vi "_Main_ByRuns_DAC2022.vi"() -> ()   [LabVIEW 2017]
uses:
  <vilib>/Instr/_visa.llb/VISA Configure Serial Port (Instr).vi
panel:
  out "Field, kV/cm":dbl
  out "Current, mA":dbl
  out "Voltage, V":dbl
  in  "COM DAC":refnum<visa-resource-name>
  in  "WaveForm":i32(listbox)
  in  "Auto\nturn OFF":bool
  in  "Content":i32(listbox)
  out "LastTrigTimer, s":dbl
  in  "Graph every, cycle":dbl=10.0 min=1.0 max=100.0
  in  "SendPeriod, ms":dbl=100.0 min=10.0 max=10000.0
  out "RunsNeed":i32
  out "Time LOG":cluster{dbl[], dbl[]}(graph)
  out "LED2":bool
  out "LED1":bool
  out "TrigTimer, s":dbl
  out "Bytes at Port":u32
  out "RecTry":i32
  out "OutVoltage, V":dbl
  in  "Exposition, s":dbl=3.0
  out "Channel 2, V":dbl format="%#_5g"
  out "Channel 1, V":dbl format="%#_5g"
  in  "Stop Button":bool
  in  "Start Button":bool
  in  "Sample H, um":dbl=32.0
  out "VoltageArray, V":dbl[](array[numeric])
  out "Shutter Red":bool
  out "Shutter Green":bool
  in  "Frames In Run":u32=180
  out "Global Frame Done":u32
  out "Now is Run #":u32
  out "Frame In Run Done":u32
  in  "Step, kV/cm":dbl=1.0 min=0.01 max=1000.0
  in  "Amplitude, kV/cm":dbl=10.0 min=10.0 max=1500.0
  in  "LOG file":path
  in  "COM ADC":refnum<visa-resource-name>
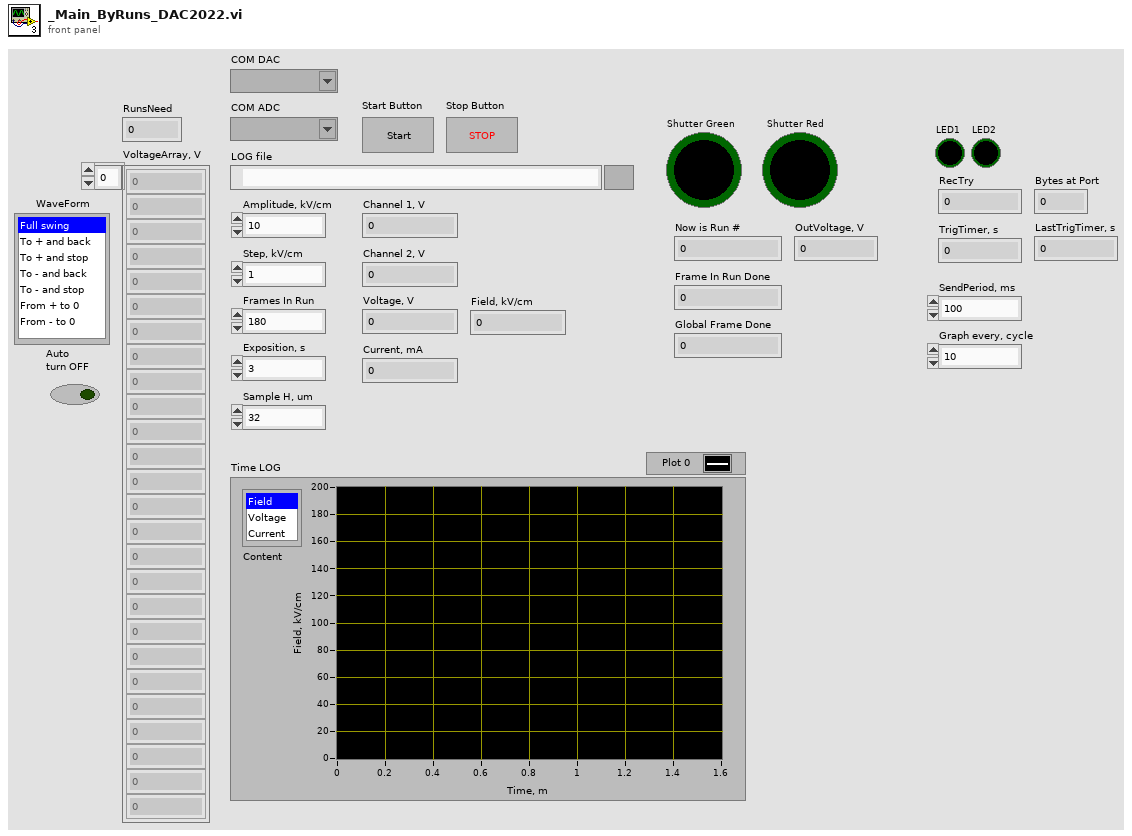
[diagram p1: front panel]
types:
  T1 = cluster{i32, i32, u32, "TrigState":bool, "TrigTimer, s":dbl, "CurrentError":bool}
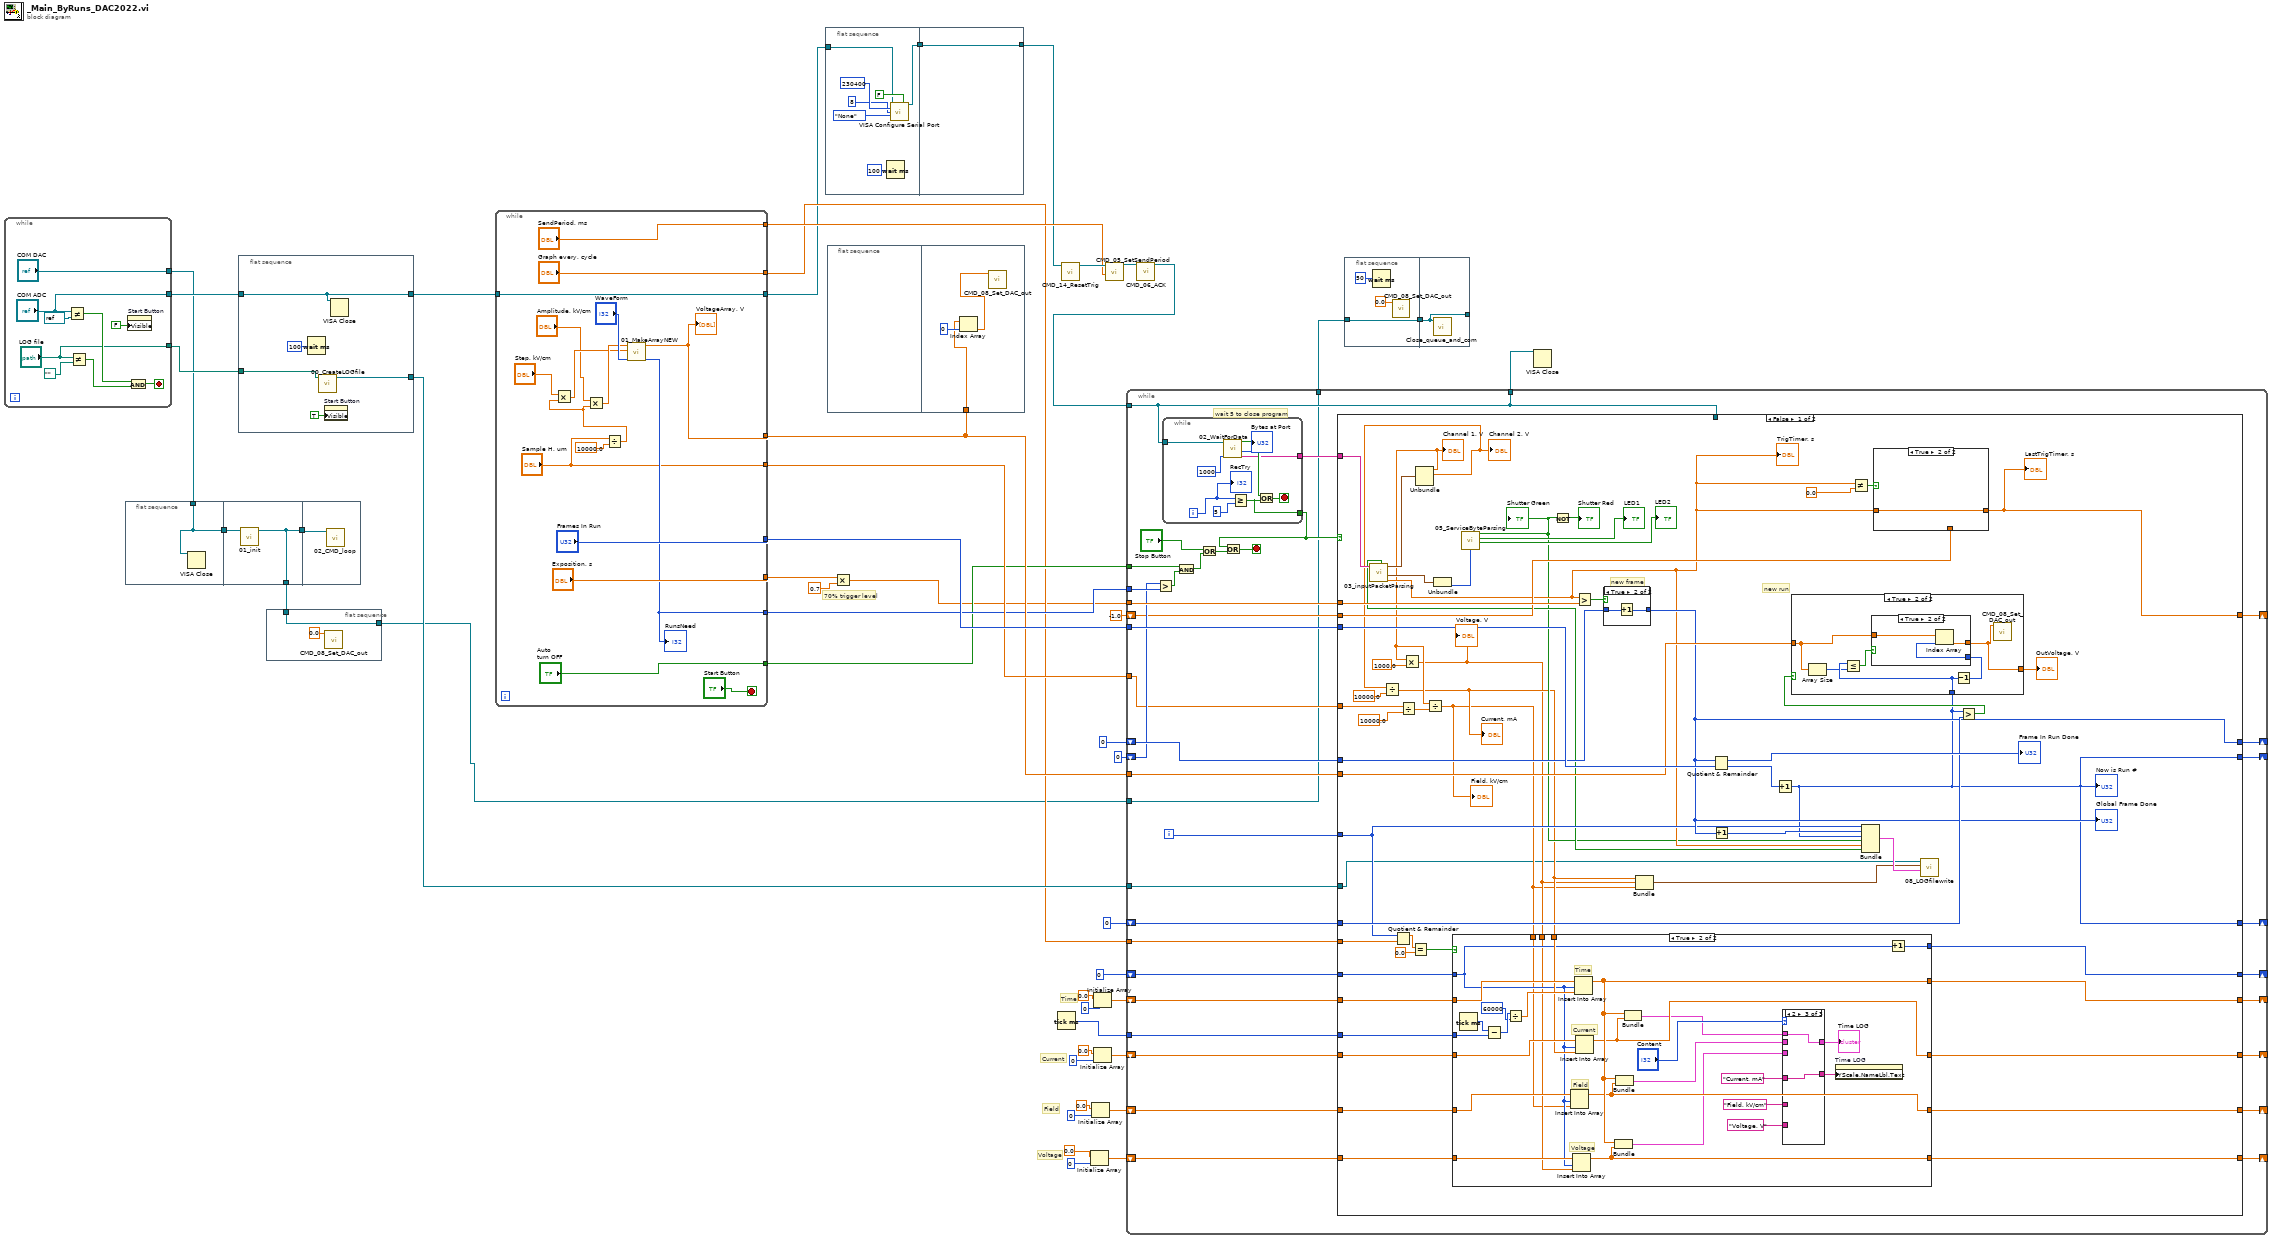
[diagram p0: block diagram]
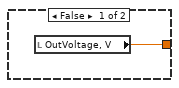
[diagram p6: hidden frame]
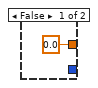
[diagram p7: hidden frame]
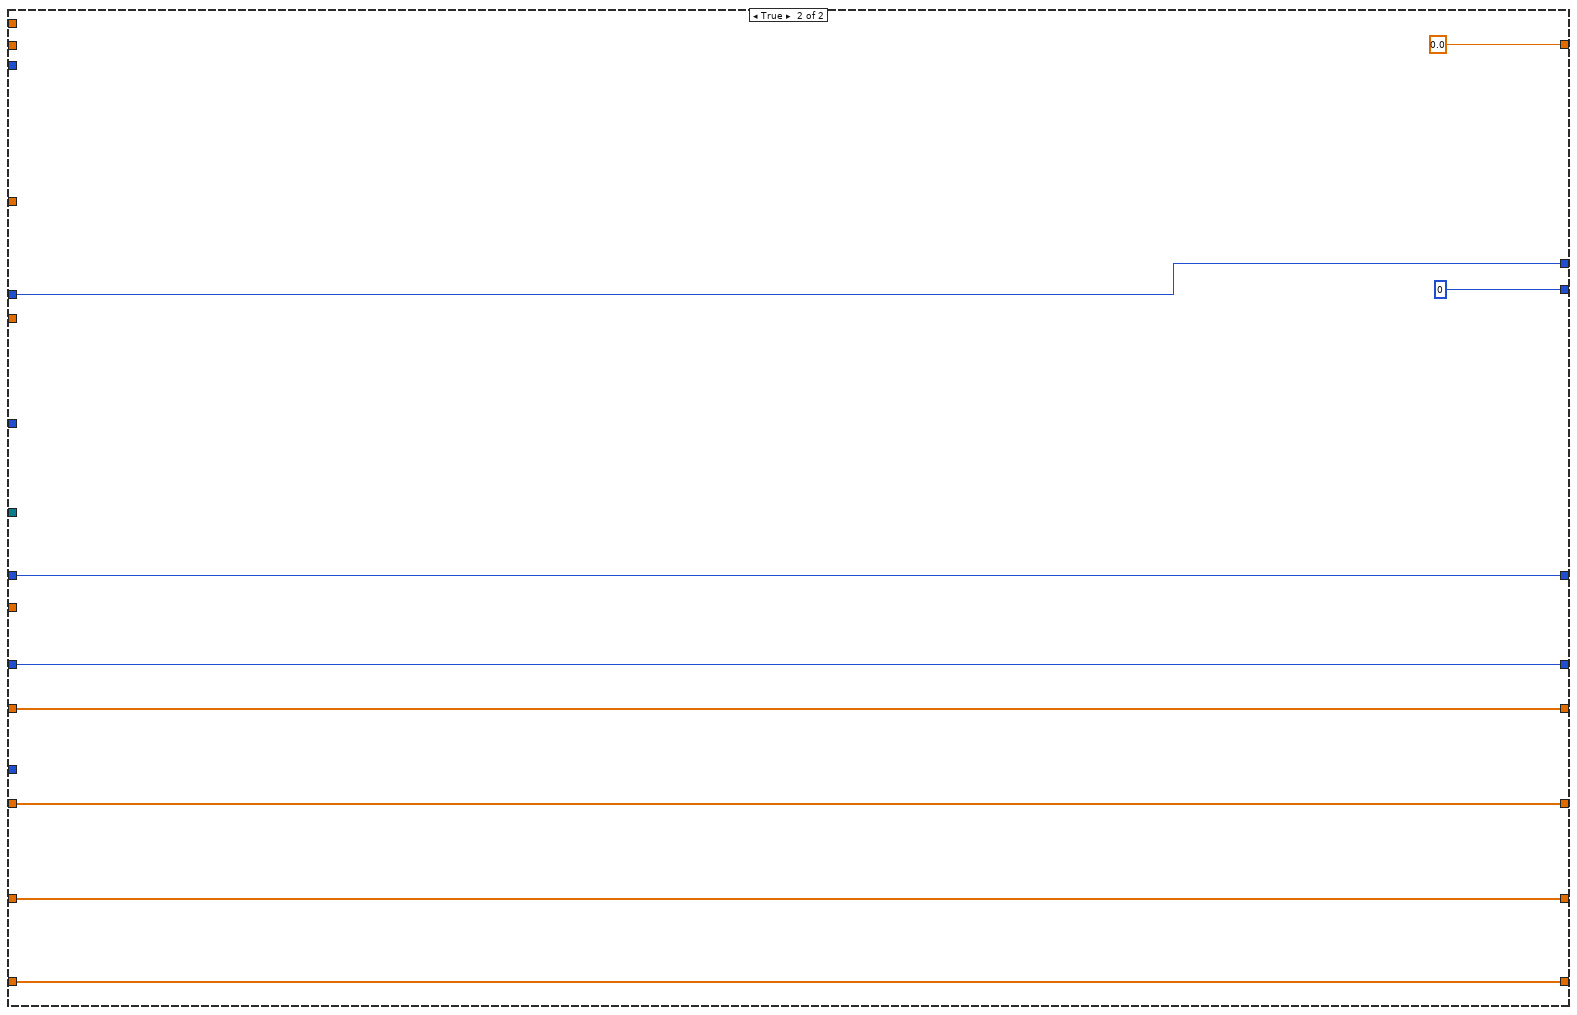
[diagram p9: hidden frame]
diagram:
  # "70% trigger level"
  # "Voltage"
  # "Field"
  # "Time"
  # "Current"
  n1 = while {
    tunnel: ["COM ADC"] -> w14
    tunnel: ["LOG file"] -> w13
    tunnel: ["COM DAC"] -> w5
    stop <- w53 stop-if-true
    n2 = Not Equal?(x="COM ADC", y=refnum<visa-resource-name> refnum ("COM port")) -> (x != y?=w50:bool)
    n3 = Not Equal?(x="LOG file", y=path "" ("LOG file")) -> (x != y?=w51:bool)
    n4 = property on="Start Button" class="Bool"("Visible"=FALSE) -> ()  [unwired: 2 in, 2 out]
    n5 = And(x=w50, y=w51) -> (x .and. y?=w53:bool)
  }
  n6 = flat-sequence {
    tunnel: [w56] -> w7
    tunnel: w5 -> [w56]
    tunnel: w7 -> [w58]
    tunnel: [w57] -> w4
    tunnel: [w57] -> w6
    tunnel: w6 -> [w59]
    frame #0 {
      n7 = VISA Close(VISA resource name=w56) -> ()  [unwired: 1 in, 1 out]
    }
    frame #1 {
      n8 = call "01_init.vi"("COM port"=w58) -> ("VISA resource name out"=w57:refnum<visa-resource-name>)  [unwired: 8 in, 2 out]
    }
    frame #2 {
      n9 = call "02_CMD_loop.vi"("VISA resource name"=w59) -> ()  [unwired: 11 in]
    }
  }
  n10 = flat-sequence {
    tunnel: [w64] -> w44
    tunnel: w14 -> [w60]
    tunnel: w13 -> [w61]
    tunnel: [w60] -> w12
    frame #0 {
      n11 = Wait (ms)(milliseconds to wait=u32 100) -> ()  [unwired: 1 out]
      n12 = call "00_CreateLOGfile.vi"("LOG file"=w61) -> ("refnum out"=w64:refnum<file>)  [unwired: 10 in]
      n13 = property on="Start Button" class="Bool"("Visible"=TRUE) -> ()  [unwired: 2 in, 2 out]
      n14 = VISA Close(VISA resource name=w60) -> ()  [unwired: 1 in, 1 out]
    }
  }
  n15 = flat-sequence {
    tunnel: w4 -> [w65]
    tunnel: [w65] -> w1
    frame #0 {
      n16 = call "CMD_08_Set_DAC_out.vi"("DAC voltage, V"=0.0) -> ()  [unwired: 11 in]
    }
  }
  n17 = while {
    tunnel: w12 -> [w76]
    tunnel: [w76] -> w10
    tunnel: [w75] -> w38
    tunnel: ["Sample H, um"] -> w45
    tunnel: ["Frames In Run"] -> w46
    tunnel: ["Exposition, s"] -> w23
    tunnel: [w74] -> w29
    tunnel: ["Auto\nturn OFF"] -> w27
    tunnel: ["SendPeriod, ms"] -> w26
    tunnel: ["Graph every, cycle"] -> w25
    stop <- "Start Button" stop-if-true
    n18 = Divide(x="Sample H, um", y=10000.0) -> (x/y=w68:dbl)
    n19 = Multiply(x="Step, kV/cm", y=w68) -> (x*y=w70:dbl)
    n20 = Multiply(x="Amplitude, kV/cm", y=w68) -> (x*y=w71:dbl)
    n21 = call "01_MakeArrayNEW.vi"("Amp"=w71, "Step"=w70, "WaveForm"="WaveForm") -> ("Array"=w75:dbl[], "ArraySize"=w74:i32)  [unwired: 6 in]
    "VoltageArray, V" <- w75
    "RunsNeed" <- w74
  }
  n22 = flat-sequence {
    tunnel: w10 -> [w86]
    tunnel: [w85] -> w11
    tunnel: w11 -> [w91]
    tunnel: [w91] -> w9
    frame #0 {
      n23 = Wait (ms)(milliseconds to wait=u32 100) -> ()  [unwired: 1 out]
      n24 = call-poly "VISA Configure Serial Port"("VISA resource name"=w86, "Enable Termination\nChar (T)"=FALSE ("Enable Termination\nChar (T)"), "baud rate (9600)"=u32 230400, "data bits (8)"=u16 8, "parity (0:none)"=enum16{"None", "Odd", "Even", "Mark", "Space"}."None") -> ("VISA resource name out"=w85:refnum<visa-resource-name>)  [unwired: 9 in, 1 out]
    }
    frame #1 {
    }
  }
  n25 = flat-sequence {
    tunnel: w38 -> [w93]
    frame #0 {
    }
    frame #1 {
      n26 = Index Array(array=w93, index=0) -> (element=w92:dbl)
      n27 = call "CMD_08_Set_DAC_out.vi"("DAC voltage, V"=w92) -> ()  [unwired: 11 in]
    }
  }
  n28 = Multiply(x=w23, y=0.7) -> (x*y=w24:dbl)
  n29 = Tick Count (ms)() -> (millisecond timer value=w33:u32)
  n30 = call "CMD_14_ResetTrig.vi"("VISA resource name"=w9) -> ("VISA resource name out"=w41:refnum<visa-resource-name>)  [unwired: 10 in]
  n31 = Initialize Array(0.0 ("element"), 0 ("dimension size")) -> (w15:dbl[])
  n32 = Initialize Array(0.0 ("element"), 0 ("dimension size")) -> (w16:dbl[])
  n33 = Initialize Array(0.0 ("element"), 0 ("dimension size")) -> (w30:dbl[])
  n34 = Initialize Array(0.0 ("element"), 0 ("dimension size")) -> (w34:dbl[])
  n35 = call "CMD_05_SetSendPeriod.vi"("Period, ms"=w26, "VISA resource name"=w41) -> ("VISA resource name out"=w40:refnum<visa-resource-name>)  [unwired: 9 in]
  n36 = call "CMD_06_ACK.vi"("VISA resource name"=w40) -> ("VISA resource name out"=w39:refnum<visa-resource-name>)  [unwired: 10 in]
  n37 = while {
    tunnel: w39 -> [w96]
    tunnel: w38 -> [w120]
    tunnel: w46 -> [w126]
    tunnel: w24 -> [w128]
    tunnel: w45 -> [w97]
    tunnel: w44 -> [w127]
    shift-right: [w123] -> _
    shift-left: 0 -> [w125]
    shift-right: [w122] -> _
    shift-left: u32 0 -> [w121]
    shift-right: [w118] -> _
    shift-left: 0 -> [w119]
    tunnel: w33 -> [w116]
    shift-right: [w114] -> _
    shift-left: w34 -> [w117]
    shift-right: [w113] -> _
    shift-left: w30 -> [w115]
    tunnel: w29 -> [w109]
    shift-right: [w111] -> _
    shift-left: u32 0 -> [w108]
    tunnel: w27 -> [w105]
    tunnel: w25 -> [w104]
    shift-right: [w103] -> _
    shift-left: -1.0 ("TrigTimer, s") -> [w102]
    shift-right: [w99] -> _
    shift-left: w16 -> [w101]
    shift-right: [w98] -> _
    shift-left: w15 -> [w100]
    tunnel: [w95] -> w2
    tunnel: [w96] -> w8
    tunnel: w1 -> [w95]
    i -> [w124]
    stop <- w131 stop-if-true
    # "wait 5 to close program"
    n38 = Greater?(x=w108, y=w109) -> (0:w106:bool)
    n39 = while {
      tunnel: w96 -> [w251]
      tunnel: [w254] -> w130
      tunnel: [w255] -> w129
      i -> [w253]
      stop <- w257 stop-if-true
      n40 = call "02_WaitForData.vi"("WaitTimeoutMS"=u32 1000, "VISA"=w251) -> ("Buffer"=w255:string, "Bytes at Port"=→"Bytes at Port":u32, "Data Recived"=w256:bool)  [unwired: 7 in]
      n41 = Greater Or Equal?(x=w253, y=5) -> (x >= y?=w254:bool)
      n42 = Or(x=w256, y=w254) -> (x .or. y?=w257:bool)
      "RecTry" <- w253
    }
    n43 = And(x=w105, y=w106) -> (x .and. y?=w107:bool)
    n44 = Or(x="Stop Button", y=w107) -> (x .or. y?=w112:bool)
    n45 = Or(x=w130, y=w112) -> (x .or. y?=w131:bool)
    n46 = case shown="False" w130 {
      tunnel: w129 -> [w187 _]
      tunnel: w128 -> [w183 _]
      tunnel: w127 -> [w132 _]
      tunnel: w126 -> [w184 _]
      tunnel: w125 -> [w181 w250]
      tunnel: w124 -> [w166 _]
      tunnel: [w173 w250] -> w123
      tunnel: [w157 w249] -> w122
      tunnel: w121 -> [w176 w249]
      tunnel: w120 -> [w177 _]
      tunnel: w96 -> [_ _]
      tunnel: w119 -> [w164 w248]
      tunnel: [w163 w248] -> w118
      tunnel: w117 -> [w162 w247]
      tunnel: w116 -> [w161 _]
      tunnel: w115 -> [w160 w246]
      tunnel: [w159 w247] -> w114
      tunnel: [w158 w246] -> w113
      tunnel: [w157 u32 0] -> w111
      tunnel: w104 -> [w156 _]
      tunnel: [w153 0.0 ("TrigTimer, s")] -> w103
      tunnel: w102 -> [w152 _]
      tunnel: w101 -> [w148 w243]
      tunnel: w100 -> [w147 w242]
      tunnel: [w146 w243] -> w99
      tunnel: [w145 w242] -> w98
      tunnel: w97 -> [w139 _]
      frame False {
        # "new run"
        # "new frame"
        n47 = call "03_inputPacketParsing.vi"("string"=w187) -> ("TrigTimer, s"=w151:dbl, "Service state"=w172:cluster{u8, u8}, "Voltage"=w185:cluster{dbl, dbl, dbl, dbl}, "CurrentError"=w150:bool)  [unwired: 6 in, 1 out]
        "TrigTimer, s" <- w151
        n48 = Quotient & Remainder(x=w166, y=w156) -> (x-y*floor(x/y)=w168:dbl)  [unwired: 1 out]
        n49 = Divide(x=w139, y=10000.0) -> (x/y=w140:dbl)
        n50 = Equal?(x=w168, y=0.0) -> (x = y?=w165:bool)
        n51 = Unbundle(w185) -> (w141:dbl, w143:dbl)  [unwired: 2 out]
        "Channel 1, V" <- w141
        "Channel 2, V" <- w143
        n52 = Divide(x=w143, y=10000.0) -> (x/y=w136:dbl)
        "Current, mA" <- w136
        n53 = Multiply(x=w141, y=1000.0) -> (x*y=w135:dbl)
        "Voltage, V" <- w135
        n54 = Divide(x=w141, y=w140) -> (x/y=w134:dbl)
        "Field, kV/cm" <- w134
        n55 = Unbundle(w172) -> (w171:u8)  [unwired: 1 out]
        n56 = case shown="True" w165 {
          tunnel: w164 -> [w194 w210]
          tunnel: [w194 w217] -> w163
          tunnel: w162 -> [w192 w215]
          tunnel: w161 -> [_ w220]
          tunnel: w160 -> [w193 w214]
          tunnel: [w193 w206] -> w158
          tunnel: [w192 w209] -> w159
          tunnel: w136 -> [_ w213]
          tunnel: w148 -> [w191 w212]
          tunnel: w147 -> [w190 w211]
          tunnel: [w191 w207] -> w146
          tunnel: [w190 w208] -> w145
          tunnel: w135 -> [_ w196]
          tunnel: w134 -> [_ w195]
          frame False {
          }
          frame True {
            # "Time"
            # "Voltage"
            # "Field"
            # "Current"
            n57 = Tick Count (ms)() -> (millisecond timer value=w221:u32)
            n58 = Subtract(x=w221, y=w220) -> (x-y=w219:u32)
            n59 = Divide(x=w219, y=u32 60000) -> (x/y=w216:dbl)
            n60 = Insert Into Array(array=w212, index=w210, new element=w195) -> (w207:dbl[])
            n61 = Insert Into Array(array=w211, index=w210, new element=w196) -> (w208:dbl[])
            n62 = Insert Into Array(array=w215, index=w210, new element=w216) -> (w209:dbl[])
            n63 = Insert Into Array(array=w214, index=w210, new element=w213) -> (w206:dbl[])
            n64 = Bundle(w209, w208) -> (w202:cluster{dbl[], dbl[]})  [unwired: 1 in]
            n65 = Bundle(w209, w207) -> (w203:cluster{dbl[], dbl[]})  [unwired: 1 in]
            n66 = Bundle(w209, w206) -> (w204:cluster{dbl[], dbl[]})  [unwired: 1 in]
            n67 = case shown="2" "Content" {
              tunnel: w204 -> [_ _ w227]
              tunnel: w203 -> [w223 _ _]
              tunnel: w202 -> [_ w225 _]
              tunnel: [w223 w225 w227] -> w201
              tunnel: "Current, mA" ("Y Scale.Name Label.Text") -> [_ _ w226]
              tunnel: "Field, kV/cm" ("Y Scale.Name Label.Text") -> [w222 _ _]
              tunnel: "Voltage, V" ("Y Scale.Name Label.Text") -> [_ w224 _]
              tunnel: [w222 w224 w226] -> w197
              frame 0, Default {
              }
              frame 1 {
              }
              frame 2 {
              }
            }
            "Time LOG" <- w201
            n68 = property on="Time LOG" class="XYGraph (strict)"("YScale.NameLbl.Text"=w197) -> ()  [unwired: 2 in, 2 out]
            n69 = Increment(x=w210) -> (x+1=w217:i32)
          }
        }
        n70 = call "05_ServiceByteParsing.vi"("InputByte"=w171) -> ("LED2"=→"LED2":bool, "LED1"=→"LED1":bool, "TrigState"=w149:bool)  [unwired: 7 in, 1 out]
        "Shutter Green" <- w149
        n71 = Not(x=w149) -> (.not. x?=→"Shutter Red":bool)
        n72 = Greater?(x=w151, y=w183) -> (0:w182:bool)
        n73 = case shown="True" w182 {
          tunnel: w181 -> [w239 w241]
          tunnel: [w239 w240] -> w173
          frame False {
          }
          frame True {
            n74 = Increment(x=w241) -> (x+1=w240:i32)
          }
        }
        "Global Frame Done" <- w173
        n75 = Bundle(w136, w135, w134) -> (w133:cluster{dbl, dbl, dbl})  [unwired: 1 in]
        n76 = Quotient & Remainder(x=w173, y=w184) -> (x-y*floor(x/y)=→"Frame In Run Done":u32, floor(x/y)=w179:u32)
        n77 = Increment(x=w173) -> (x+1=w174:i32)
        n78 = Increment(x=w179) -> (x+1=w157:u32)
        "Now is Run #" <- w157
        n79 = Not Equal?(x=w151, y=0.0) -> (x != y?=w155:bool)
        n80 = Bundle(w166, w174, w157, "TrigState"=w149, "TrigTimer, s"=w151, "CurrentError"=w150) -> (w137:T1)  [unwired: 1 in]
        n81 = case shown="True" w155 {
          tunnel: [w188 w189] -> w153
          tunnel: w151 -> [_ w189]
          tunnel: w152 -> [w188 _]
          frame False {
          }
          frame True {
          }
        }
        "LastTrigTimer, s" <- w153
        n82 = call "08_LOGfilewrite.vi"("Counters"=w137, "output cluster"=w133, "refnum out"=w132) -> ()  [unwired: 9 in]
        n83 = Greater?(x=w157, y=w176) -> (0:w180:bool)
        n84 = case shown="True" w180 {
          tunnel: w177 -> [_ w230]
          tunnel: w157 -> [_ w233]
          tunnel: [w228 w229] -> w175
          frame False {
            n85 = local read "OutVoltage, V"() -> (w228:dbl)
          }
          frame True {
            n86 = Array Size(array=w230) -> (size(s)=w232:i32)
            n87 = Less Or Equal?(x=w233, y=w232) -> (x <= y?=w231:bool)
            n88 = Decrement(x=w233) -> (x-1=w234:u32)
            n89 = case shown="True" w231 {
              tunnel: w234 -> [_ w238]
              tunnel: w230 -> [_ w237]
              tunnel: [0.0 w236] -> w229
              frame False {
              }
              frame True {
                n90 = Index Array(array=w237, index=w238) -> (element=w236:dbl)
              }
            }
            n91 = call "CMD_08_Set_DAC_out.vi"("DAC voltage, V"=w229) -> ()  [unwired: 11 in]
          }
        }
        "OutVoltage, V" <- w175
      }
      frame True {
      }
    }
  }
  n92 = flat-sequence {
    tunnel: w2 -> [w261]
    tunnel: [w261] -> w3
    tunnel: [w263] -> _
    tunnel: w3 -> [w263]
    frame #0 {
      n93 = Wait (ms)(milliseconds to wait=u32 50) -> ()  [unwired: 1 out]
      n94 = call "CMD_08_Set_DAC_out.vi"("DAC voltage, V"=0.0) -> ()  [unwired: 11 in]
    }
    frame #1 {
      n95 = call "Close_queue_and_com.vi"("VISA"=w263) -> ()  [unwired: 11 in]
    }
  }
  n96 = VISA Close(VISA resource name=w8) -> ()  [unwired: 1 in, 1 out]
